vi "init.vi"(8 "error in (no error)":errorcluster, 11 "VISA resource name":refnum<visa-resource-name>="COM9") -> (0 "error out":errorcluster={"status"=FALSE, "code"=1073676294, "source"="VISA Read in rad_init.vi"}, 2 "read buffer":string="\r\nLaser control for ATMega128 ver. 1.90\r\nProgram ROM control sum= 19924007\r\nBoot ROM control sum= 408173\r\nControl to PC\r\n", 3 "VISA resource name out":refnum<visa-resource-name>="COM9")   [LabVIEW 2017, in "radiant.lvlib"]
doc: "<B>Laser Goto with FCU</B> VI tunes laser to the position <B>Wavenumber (1/cm)</B>. FCU1 is adjusted accordingly."
uses:
  <vilib>/Instr/_visa.llb/VISA Configure Serial Port (Instr).vi
  radiant.lvlib
panel:
  out "Numeric":i32=11
  out "bytes":u32
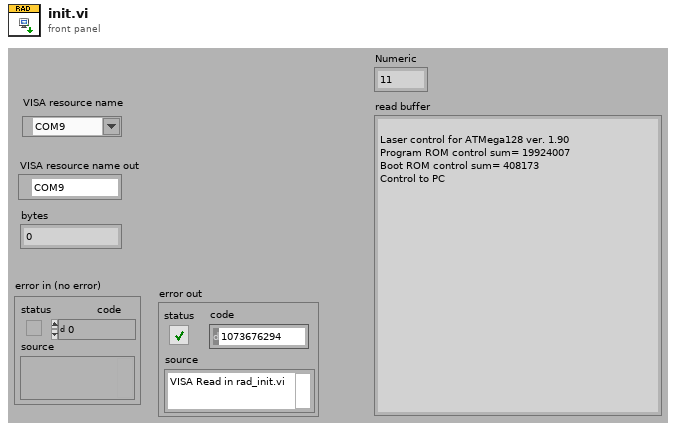
[diagram p1: front panel]
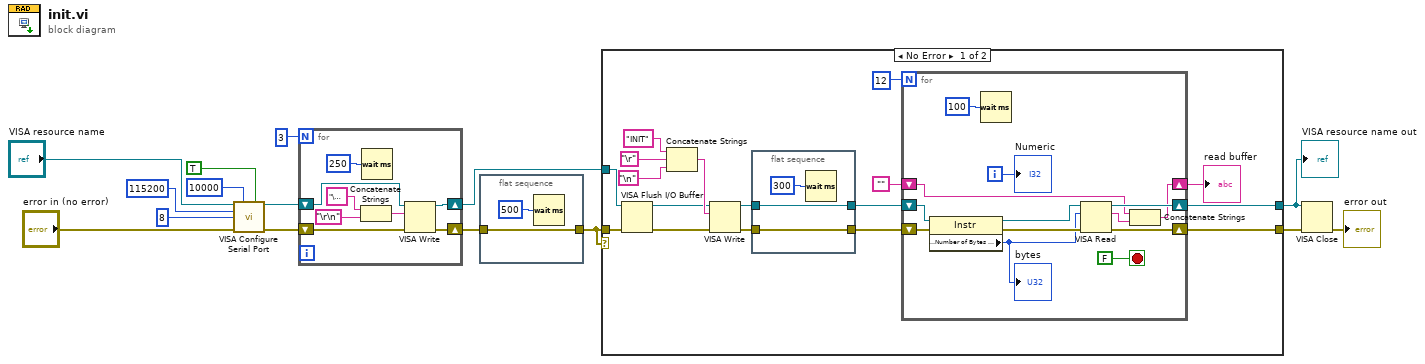
[diagram p0: block diagram]
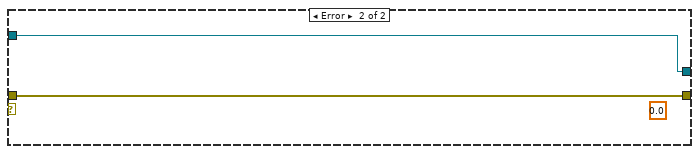
[diagram p2: hidden frame]
diagram:
  n1 = call-poly "VISA Configure Serial Port"("VISA resource name"="VISA resource name", "timeout (10sec)"=u32 10000, "Enable Termination\nChar (T)"=TRUE ("Enable Termination\nChar (T)"), "baud rate (9600)"=u32 115200, "data bits (8)"=u16 8, "error in (no error)"="error in (no error)") -> ("VISA resource name out"=w5:refnum<visa-resource-name>, "error out"=w1:errorcluster)  [unwired: 8 in]
  n2 = for {
    N: 3 -> [_]
    shift-right: [w19] -> w6
    shift-left: w1 -> [w18]
    shift-right: [w16] -> w4
    shift-left: w5 -> [w17]
    n3 = Concatenate Strings("\u001b" ("write buffer"), "\r\n") -> (w22:string)
    n4 = Wait (ms)(milliseconds to wait=u32 250) -> ()  [unwired: 1 out]
    n5 = VISA Write(VISA resource name=w17, write buffer=w22, error in (no error)=w18) -> (VISA resource name out=w16:refnum<visa-resource-name>, error out=w19:errorcluster)  [unwired: 1 out]
  }
  n6 = flat-sequence {
    tunnel: w6 -> [w24]
    tunnel: [w24] -> w3
    frame #0 {
      n7 = Wait (ms)(milliseconds to wait=u32 500) -> ()  [unwired: 1 out]
    }
  }
  n8 = case shown="No Error" w3 {
    tunnel: w3 -> [w38 w60]
    tunnel: w4 -> [w37 w59]
    tunnel: [w34 w60] -> w11
    tunnel: [w33 w59] -> w10
    frame No Error {
      n9 = VISA Flush I/O Buffer(VISA resource name=w37, error in (no error)=w38) -> (VISA resource name out=w36:refnum<visa-resource-name>, error out=w35:errorcluster)  [unwired: 1 in]
      n10 = Concatenate Strings("INIT" ("write"), "\r", "\n") -> (w39:string)
      n11 = VISA Write(VISA resource name=w36, write buffer=w39, error in (no error)=w35) -> (VISA resource name out=w32:refnum<visa-resource-name>, error out=w31:errorcluster)  [unwired: 1 out]
      n12 = flat-sequence {
        tunnel: w32 -> [w58]
        tunnel: [w58] -> w29
        tunnel: w31 -> [w57]
        tunnel: [w57] -> w30
        frame #0 {
          n13 = Wait (ms)(milliseconds to wait=u32 300) -> ()  [unwired: 1 out]
        }
      }
      n14 = for {
        N: 12 -> [_]
        shift-right: [w55] -> w34
        shift-left: w30 -> [w51]
        shift-right: [w54] -> w33
        shift-left: w29 -> [w50]
        shift-right: [w45] -> w26
        shift-left: "" -> [w48]
        i -> [w46]
        stop <- FALSE stop-if-true
        n15 = property class="Instr"(reference=w50, error in=w51) -> (reference out=w53:refnum<visa-resource-name>, error out=w52:errorcluster, "Serial Settings:Number of Bytes at Serial Port"=w44:u32)
        "bytes" <- w44
        n16 = Wait (ms)(milliseconds to wait=u32 100) -> ()  [unwired: 1 out]
        n17 = VISA Read(VISA resource name=w53, byte count=w44, error in (no error)=w52) -> (VISA resource name out=w54:refnum<visa-resource-name>, read buffer=w49:string, error out=w55:errorcluster)  [unwired: 1 out]
        n18 = Concatenate Strings(w48, w49) -> (w45:string)
        "Numeric" <- w46
      }
      "read buffer" <- w26
    }
    frame Error {
      (unwired) 0.0
    }
  }
  "VISA resource name out" <- w10
  n19 = VISA Close(VISA resource name=w10, error in (no error)=w11) -> (error out=→"error out":errorcluster)
